vi "erroOut.vi"(9 "source":string, 10 "code":i32) -> (2 "output cluster":errorcluster)   [LabVIEW 2025, in "tcv.lvlib" / "tcv.lvclass"]
uses:
  tcv/tcv.lvclass
  tcv/tcv.lvclass/tcv.ctl
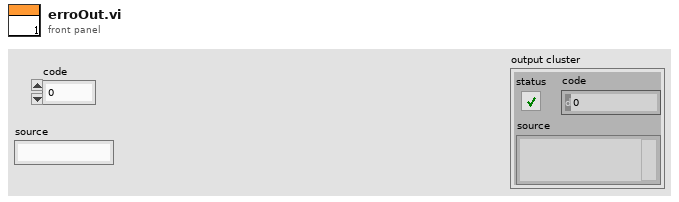
[diagram p1: front panel]
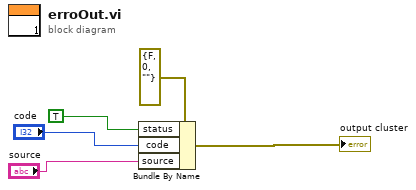
[diagram p0: block diagram]
diagram:
  n1 = Bundle By Name(cluster=errorcluster {"status"=FALSE, "code"=0, "source"=""} ("error in"), "status"=TRUE, "code"="code", "source"="source") -> (→"output cluster":errorcluster)
